vi "Get All Keys and Values.vi"(8 "error in":errorcluster, 11 "JSON Value in":refnum<class "JSON Value.lvclass">) -> (0 "error out":errorcluster, 1 "values":refnum<class "JSON Value.lvclass">[](array[class]), 2 "keys":string[](array[string]))   [LabVIEW 2016, in "JSON Value.lvclass"]
doc: "Returns an array of all of the keys and an array of their corresponding values. Elements are correlated by index, so the key at a given index corresponds to the value at the same index."
uses:
  JSON Value.lvclass
  JSON Value.lvclass/JSON Value.ctl
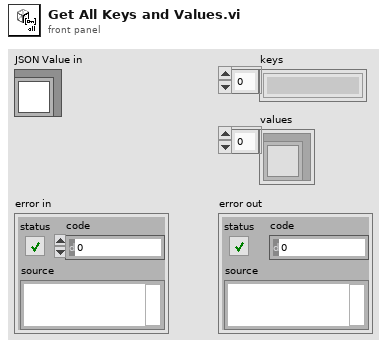
[diagram p1: front panel]
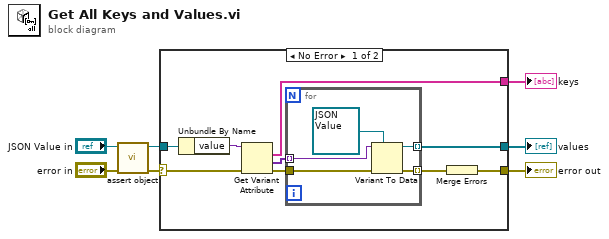
[diagram p0: block diagram]
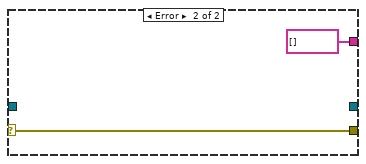
[diagram p2: hidden frame]
diagram:
  n1 = call "assert object.vi"("error in (no error)"="error in", "JSON Value in"="JSON Value in") -> ("error out"=w3:errorcluster, "JSON Value out"=w1:refnum<class "JSON Value.lvclass">)  [unwired: 8 in]
  n2 = case shown="No Error" w3 {
    selector: w3 -> [w12 w23]
    tunnel: [w14 string[] []] -> w7
    tunnel: [w13 _] -> w6
    tunnel: [w10 w23] -> w4
    tunnel: w1 -> [w11 _]
    frame No Error {
      n3 = Unbundle By Name(w11) -> ("value"=w16:variant)
      n4 = Get Variant Attribute(Variant=w16, error in=w12) -> (names=w14:string[], values=w15:variant[], error out=w8:errorcluster)  [unwired: 2 in, 1 out]
      n5 = for {
        tunnel: w15 -> [w21] mode=indexing
        tunnel: [w20] -> w13 mode=indexing
        tunnel: [w19] -> w9 mode=indexing
        tunnel: w8 -> [w18]
        n6 = Variant To Data(error in=w18, type=refnum<class "JSON Value.lvclass"> refnum ("JSON Object in"), Variant=w21) -> (data=w20:refnum<class "JSON Value.lvclass">, error out=w19:errorcluster)
      }
      n7 = Merge Errors(w9) -> (w10:errorcluster)
    }
    frame Error {
    }
  }
  "keys" <- w7
  "values" <- w6
  "error out" <- w4
